vi "RemoveChildFromNode.vi"(8 "error in":errorcluster, 10 "removed child":T1, 11 "NISE_CEF_serializable node folder in":refnum<class "NISE_CEF_serializable node folder.lvclass">) -> (0 "error out":errorcluster, 3 "NISE_CEF_serializable node folder out":refnum<class "NISE_CEF_serializable node folder.lvclass">)   [LabVIEW 2013, in "NISE_CEF_serializable node folder.lvclass"]
uses:
  NISE_CEF_serializable node folder.lvclass
  Node/NodeRef.ctl
  Node/NISE_CEF_Node.lvclass
  serializable node/NISE_CEF_serializable node.lvclass
  Node/NISE_CEF_Node.lvclass/NISE_CEF_Node.ctl
  Node/ReadParent.vi
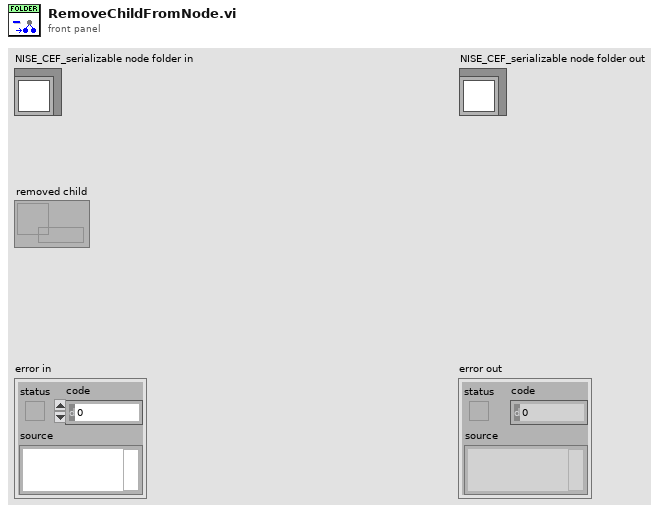
[diagram p1: front panel]
types:
  T1 = typedef "NISE_CEF_Node.lvclass/NodeRef.ctl" = refnum<data-value>
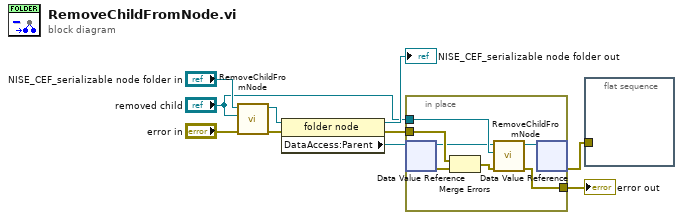
[diagram p0: block diagram]
diagram:
  n1 = call-parent "RemoveChildFromNode.vi"("error in"="error in", "removed child"="removed child", "NISE_CEF_Node in"="NISE_CEF_serializable node folder in") -> ("error out"=w10:errorcluster, "NISE_CEF_Node out"=w7:refnum<class "NISE_CEF_serializable node folder.lvclass">)  [unwired: 7 in]
  n2 = property class="folder node"(reference=w7, error in=w10) -> (reference out=→"NISE_CEF_serializable node folder out":refnum<class "NISE_CEF_serializable node folder.lvclass">, error out=w5:errorcluster, "DataAccess:Parent"=w2:T1)
  n3 = in-place {
    in-place-border: w5 -> [w17]
    in-place-border: [w16] -> w4
    in-place-border: "removed child" -> [w15]
    n4 = in-place-dvr #1(w2) -> (w14:refnum<class "NISE_CEF_Node.lvclass">, w11:errorcluster)
    n5 = Merge Errors(w17, w11) -> (w12:errorcluster)
    n6 = call-dynamic "RemoveChildFromNode.vi"("error in"=w12, "removed child"=w15, "NISE_CEF_Node in"=w14) -> ("error out"=w16:errorcluster, "NISE_CEF_Node out"=w13:refnum<class "NISE_CEF_Node.lvclass">)  [unwired: 7 in]
    n7 = in-place-dvr #1(w13) -> (w1:errorcluster)  [unwired: 1 out]
  }
  "error out" <- w4
  n8 = flat-sequence {
    tunnel: w1 -> [_]
    frame #0 {
    }
  }
